vi "Get Class Name.vi"(1 "Elite DAQ Board in":refnum<class "Elite DAQ Design.lvclass">) -> (0 "class name":string)   [LabVIEW 2023, in "Elite DAQ Design.lvclass"]
doc: "Get the name of this class."
uses:
  Elite DAQ Design.lvclass
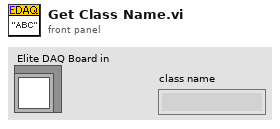
[diagram p1: front panel]
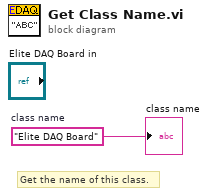
[diagram p0: block diagram]
diagram:
  w1 = "Elite DAQ Board"  # class name
  # "Get the name of this class."
  "class name" <- w1
